vi "Read Input Events.vi"(8 "error in (no error)":errorcluster, 11 "Parameters in":refnum<class "Parameters.lvclass">) -> (0 "error out":errorcluster, 2 "Input Events":T1[](array[typedef]), 3 "Parameters out":refnum<class "Parameters.lvclass">)   [LabVIEW 2020, in "Parameters.lvclass"]
uses:
  Parameters.lvclass
  Digital Input VIs/Tosca-Input Event.ctl
  Digital Input VIs/Tosca-Input Criterion.ctl
  epl-vi-lib/Utility VIs/Type Defs/Logic State.ctl
  Typedefs/Tosca-Accumulator.ctl
  Parameters.lvclass/Parameters.ctl
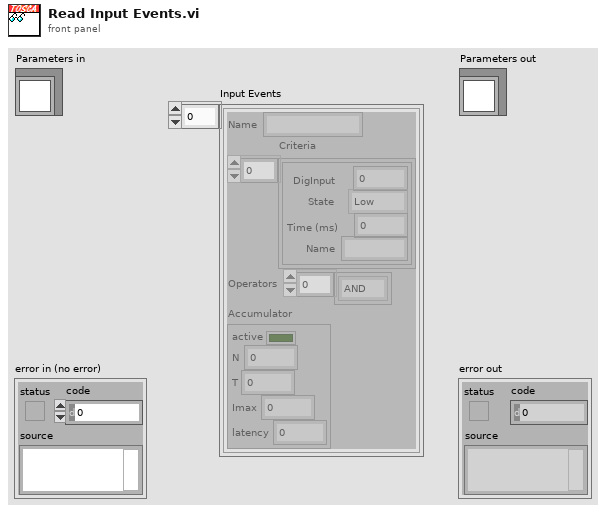
[diagram p1: front panel]
types:
  T1 = typedef "Tosca-Input Event.ctl" = cluster{"Name":string, "Criteria":T2[], "Operators":enum16{"AND", "OR"}[], "Accumulator":T4}
  T2 = typedef "Tosca-Input Criterion.ctl" = cluster{"DigInput":i32, "State":T3, "Time (ms)":i32, "Name":string}
  T3 = typedef "Logic State.ctl" = enum16{"Low", "High", "Rising", "Falling"}
  T4 = typedef "Tosca-Accumulator.ctl" = cluster{"active":bool, "N":i32, "T":dbl, "Imax":dbl, "latency":dbl}
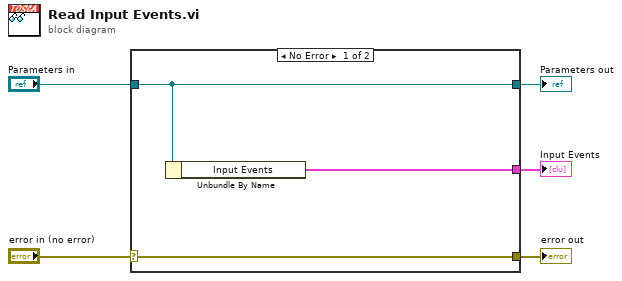
[diagram p0: block diagram]
diagram:
  n1 = case shown="No Error" "error in (no error)" {
    selector: "error in (no error)" -> [w8 w9]
    tunnel: [w8 w9] -> w4
    tunnel: [w7 w10] -> w2
    tunnel: "Parameters in" -> [w7 w10]
    tunnel: [w6 _] -> w1
    frame No Error {
      n2 = Unbundle By Name(w7) -> ("Input Events"=w6:T1[])
    }
    frame Error {
    }
  }
  "error out" <- w4
  "Parameters out" <- w2
  "Input Events" <- w1
